vi "LinearSystemId_IdentifyVelocitySystem.vi"(10 "kA":dbl, 11 "kV":dbl) -> (3 "Linearsystem":T1)   [LabVIEW 2019, in "Trajectory_Library.lvlib"]
doc: "Creates a new LINEAR SYSTEM data cluster with the specified values. \n\n\nInputs: \n - XXX -- XXX.\n\nOutputs:\n - XXX -- XXX."
uses:
  Trajectory_Library.lvlib
  LINEAR_SYSTEM.ctl
  MatrixHelper_CoerceSize.vi
  <vilib>/Analysis/Matrix/Datatypes/RealMatrix.ctl
  <vilib>/Analysis/Matrix/NI_Matrix.lvlib
panel:
  in  "Outputs":i32=1
  in  "Inputs":i32=1
  in  "States":i32=1
  # "<States,States>"
  # "<States,Inputs>"
  # "<Outputs,States>"
  # "<Outputs,Inputs>"
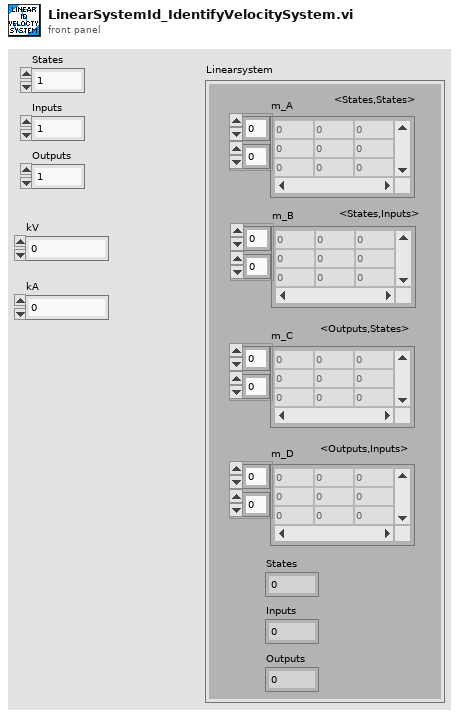
[diagram p1: front panel]
types:
  T1 = typedef "Trajectory_Library.lvlib/LINEAR_SYSTEM.ctl" = cluster{"m_A":T2, "m_B":T2, "m_C":T2, "m_D":T2, "States":i32, "Inputs":i32, "Outputs":i32}
  T2 = typedef "NI_Matrix.lvlib/RealMatrix.ctl" = dbl[][]
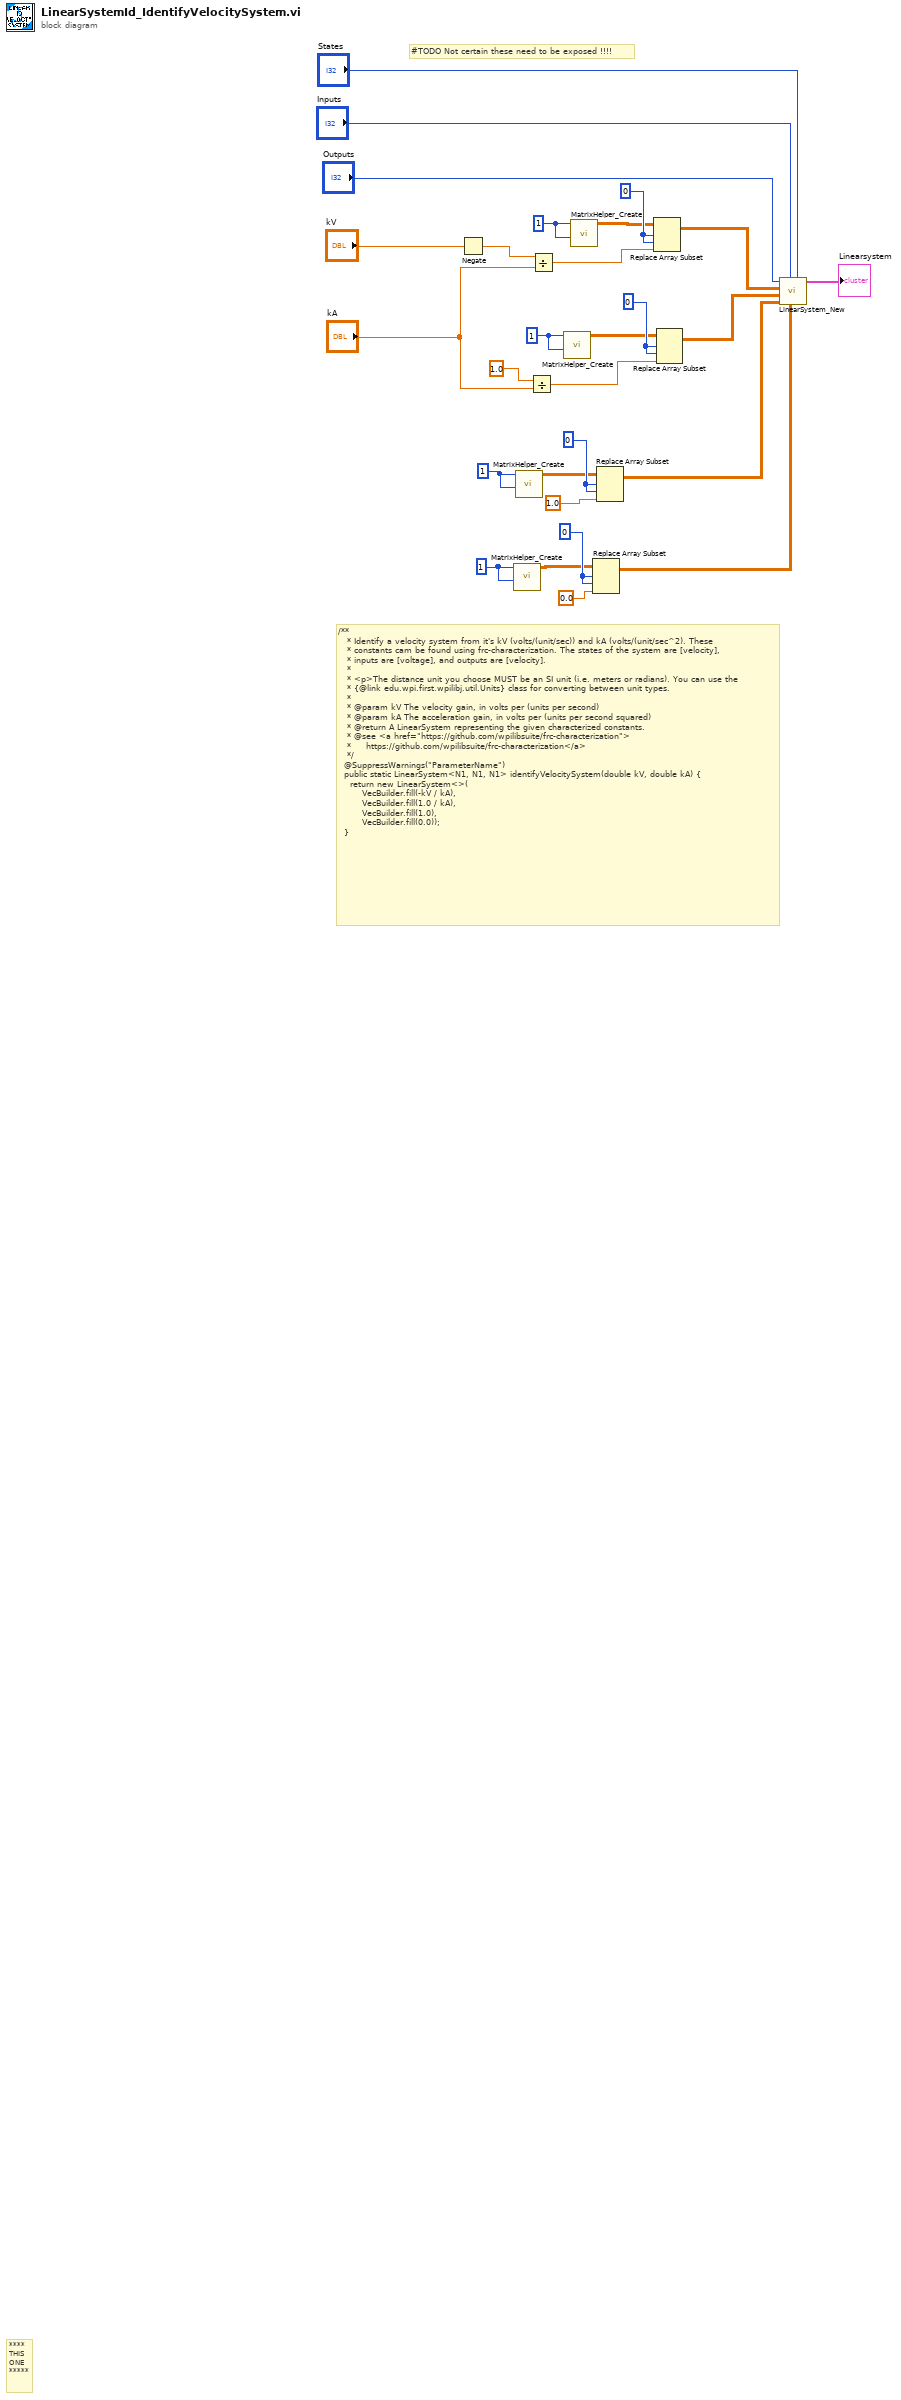
[diagram p0: block diagram]
diagram:
  w2 = 1 ("number of rows")
  w4 = 1 ("number of rows")
  w6 = 1 ("number of rows")
  w16 = 0 ("index (col)")
  w18 = 0 ("index (col)")
  w22 = 0 ("index (col)")
  w24 = 0 ("index (col)")
  w8 = 1 ("number of rows")
  # "#TODO Not certain these need to be exposed !!!!"
  # "/**\n   * Identify a velocity system from it's kV (volts/(unit/sec)) and kA (volts/(unit/sec^2). These\n   * constants cam be found using frc-characterization. The states of the system are [velocity],\n   * inputs are [voltage], and outputs are [velocity].\n   *\n   * <p>The distance unit you choose MUST be an SI unit (i.e. meters or radians). You can use the\n   * {@link edu.wpi.first.wpilibj.util.Units} class for converting between unit types.\n   *\n   * @param kV The velocity gain, in volts per (units per second)\n   * @param kA The acceleration gain, in volts per (units per second squared)\n   * @return A LinearSystem representing the given characterized constants.\n   * @see <a href=\"https://github.com/wpilibsuite/frc-characterization\">\n   *     https://github.com/wpilibsuite/frc-characterization</a>\n   */\n  @SuppressWarnings(\"ParameterName\")\n  public static LinearSystem<N1, N1, N1> identifyVelocitySystem(double kV, double kA) {\n    return new LinearSystem<>(\n        VecBuilder.fill(-kV / kA),\n        VecBuilder.fill(1.0 / kA),\n        VecBuilder.fill(1.0),\n        VecBuilder.fill(0.0));\n  }"
  # "****\nTHIS\nONE\n*****"
  n1 = Negate(x="kV") -> (-x=w12:dbl)
  n2 = call "MatrixHelper_Create.vi"("Columns"=w8, "Rows"=w8) -> ("output matrix"=w7:T2)  [unwired: 9 in]
  n3 = call "MatrixHelper_Create.vi"("Columns"=w6, "Rows"=w6) -> ("output matrix"=w5:T2)  [unwired: 9 in]
  n4 = Divide(x=1.0, y="kA") -> (x/y=w21:dbl)
  n5 = Divide(x=w12, y="kA") -> (x/y=w23:dbl)
  n6 = call "MatrixHelper_Create.vi"("Columns"=w4, "Rows"=w4) -> ("output matrix"=w3:T2)  [unwired: 9 in]
  n7 = call "MatrixHelper_Create.vi"("Columns"=w2, "Rows"=w2) -> ("output matrix"=w1:T2)  [unwired: 9 in]
  n8 = Replace Array Subset(array=w7, new element=0.0 ("new element/submatrix"), index (row)=w18, index (col)=w18) -> (w17:T2)
  n9 = Replace Array Subset(array=w5, new element=1.0 ("new element/submatrix"), index (row)=w16, index (col)=w16) -> (w15:T2)
  n10 = Replace Array Subset(array=w1, new element=w23, index (row)=w24, index (col)=w24) -> (w20:T2)
  n11 = Replace Array Subset(array=w3, new element=w21, index (row)=w22, index (col)=w22) -> (w19:T2)
  n12 = call "LinearSystem_New.vi"("States"="States", "D"=w17, "Inputs"="Inputs", "C"=w15, "B"=w19, "A"=w20, "Outputs"="Outputs") -> ("Linearsystem"=→"Linearsystem":T1)  [unwired: 4 in]
